vi "Calculate Relative Click Location.vi"(8 "Click Vertical Position":i32, 9 "Cell Top Position":i32, 10 "Cell Height":i32, 11 "Tree Click Interpreter in":refnum<class "Tree Click Interpreter.lvclass">) -> (2 "Relative Click Location":T1, 3 "Tree Click Interpreter out":refnum<class "Tree Click Interpreter.lvclass">)   [LabVIEW 2017, in "Tree Click Interpreter.lvclass"]
uses:
  <vilib>/gpm_packages/@cs/Test-executive-builder/Source/Test Executive Builder View/Tree Click Interpreter/Tree Click Interpreter.lvclass
  <vilib>/gpm_packages/@cs/Test-executive-builder/Source/Application Dependencies/Relative Click Location.ctl
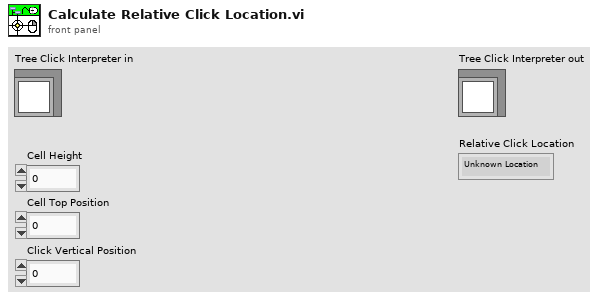
[diagram p1: front panel]
types:
  T1 = typedef "Relative Click Location.ctl" = enum16{"Unknown Location", "Below Element", "On Element", "Above Element"}
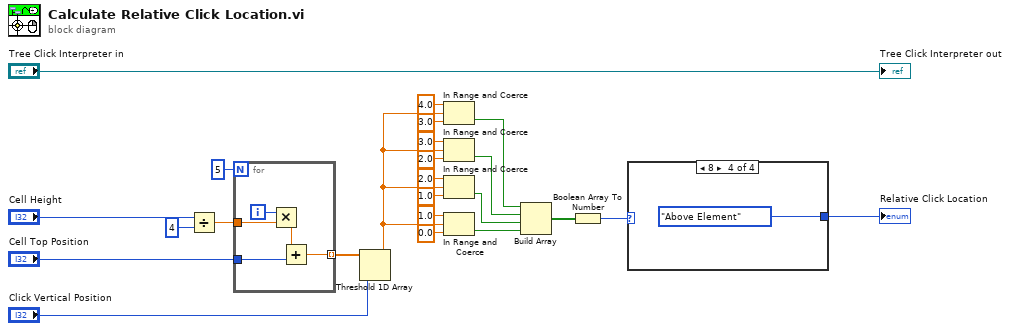
[diagram p0: block diagram]
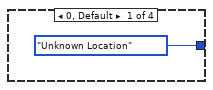
[diagram p2: hidden frame]
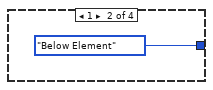
[diagram p3: hidden frame]
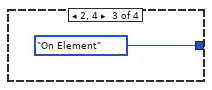
[diagram p4: hidden frame]
diagram:
  n1 = Divide(x="Cell Height", y=4 ("Cell Height")) -> (x/y=w20:dbl)
  n2 = for {
    N: 5 -> [_]
    tunnel: w20 -> [w29]
    tunnel: "Cell Top Position" -> [w27]
    tunnel: [w25] -> w18 mode=indexing
    i -> [w28]
    n3 = Multiply(x=w28, y=w29) -> (x*y=w26:dbl)
    n4 = Add(x=w26, y=w27) -> (x+y=w25:dbl)
  }
  n5 = Threshold 1D Array(2:"Click Vertical Position", 3:w18) -> (0:w8:dbl)  [unwired: 1 in]
  n6 = In Range and Coerce(upper limit=4.0, x=w8, lower limit=3.0) -> (In Range?=w4:bool)  [unwired: 1 out]
  n7 = In Range and Coerce(upper limit=3.0, x=w8, lower limit=2.0) -> (In Range?=w5:bool)  [unwired: 1 out]
  n8 = In Range and Coerce(upper limit=2.0, x=w8, lower limit=1.0) -> (In Range?=w6:bool)  [unwired: 1 out]
  n9 = In Range and Coerce(upper limit=1.0, x=w8, lower limit=0.0) -> (In Range?=w7:bool)  [unwired: 1 out]
  n10 = Build Array(w4, w5, w6, w7) -> (w3:bool[])
  n11 = Boolean Array To Number(Boolean array=w3) -> (number=w2:u32)
  n12 = case shown="8" w2 {
    tunnel: [Relative_Click_Location."Unknown Location" ("Relative Click Location") Relative_Click_Location."Below Element" ("Relative Click Location") Relative_Click_Location."On Element" ("Relative Click Location") Relative_Click_Location."Above Element" ("Relative Click Location")] -> w1
    frame 0, Default {
    }
    frame 1 {
    }
    frame 2, 4 {
    }
    frame 8 {
    }
  }
  "Relative Click Location" <- w1
  "Tree Click Interpreter out" <- "Tree Click Interpreter in"
